vi "SigMath Class - Set FP Window Title.vi"(5 "error in (no error)":errorcluster, 7 "Application Name":string="Unknown") -> (19 "error out":errorcluster)   [LabVIEW 2020, in "SigMath.lvclass"]
uses:
  SigMath.lvclass
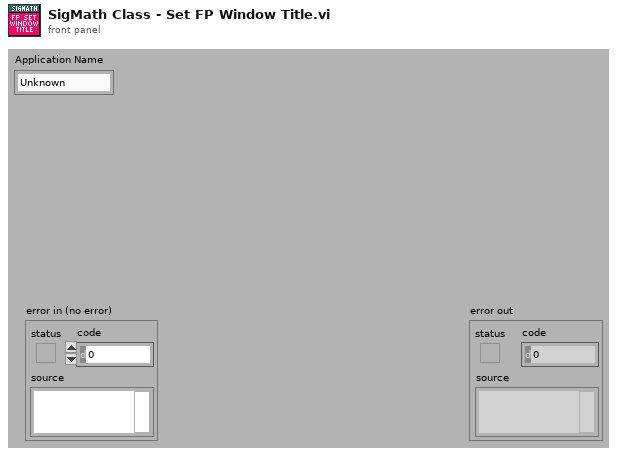
[diagram p1: front panel]
types:
  T1 = typedef "SigMath.lvclass/ClassAttributes.ctl" = cluster{"Window List":refnum<vi>[]}
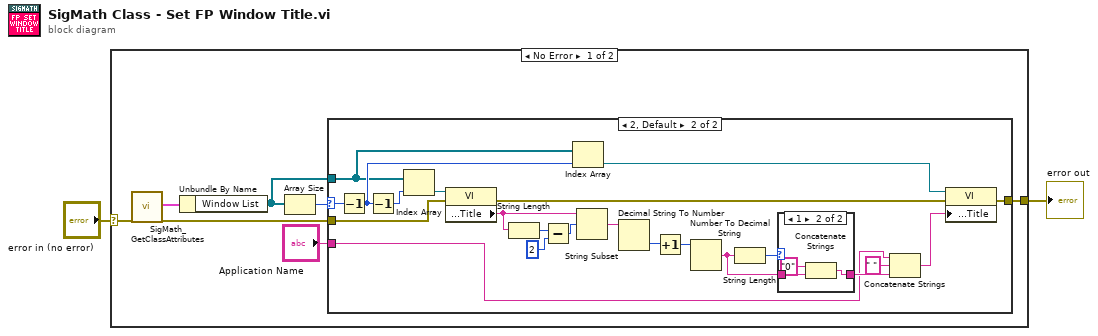
[diagram p0: block diagram]
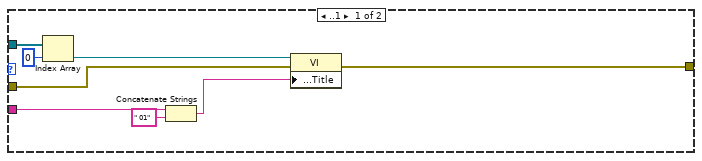
[diagram p2: hidden frame]
diagram:
  n1 = case shown="No Error" "error in (no error)" {
    selector: "error in (no error)" -> [w9 w44]
    tunnel: [w4 w44] -> w1
    frame No Error {
      n2 = call "SigMath_GetClassAttributes.vi"("error in (no error)"=w9) -> ("class attributes"=w8:T1, "error out"=w5:errorcluster)  [unwired: 15 in, 2 out]
      n3 = Unbundle By Name(w8) -> ("Window List"=w6:refnum<vi>[])
      n4 = Array Size(array=w6) -> (size(s)=w7:i32)
      n5 = case shown="2, Default" w7 {
        selector: w7 -> [_ w39]
        tunnel: w6 -> [w17 w34]
        tunnel: w5 -> [w13 w36]
        tunnel: [w14 w31] -> w4
        tunnel: "Application Name" -> [w12 w19]
        frame ..1 {
          n6 = Index Array(array=w17, index=0) -> (element=w15:refnum<vi>)
          n7 = Concatenate Strings(w12, " 01" ("string")) -> (w10:string)
          n8 = property class="VI"(reference=w15, error in=w13, "Front Panel.Title"=w10) -> (error out=w14:errorcluster)  [unwired: 1 out]
        }
        frame 2, Default {
          n9 = Decrement(x=w39) -> (x-1=w35:i32)
          n10 = Decrement(x=w35) -> (x-1=w38:i32)
          n11 = Index Array(array=w34, index=w38) -> (element=w37:refnum<vi>)
          n12 = property class="VI"(reference=w37, error in=w36) -> (error out=w33:errorcluster, "Front Panel.Title"=w30:string)  [unwired: 1 out]
          n13 = String Length(string=w30) -> (length=w29:i32)
          n14 = Subtract(x=w29, y=2) -> (x-y=w27:i32)
          n15 = Index Array(array=w34, index=w35) -> (element=w32:refnum<vi>)
          n16 = String Subset(string=w30, offset (0)=w27) -> (substring=w26:string)  [unwired: 1 in]
          n17 = Decimal String To Number(string=w26) -> (number=w25:i32)  [unwired: 2 in, 1 out]
          n18 = Increment(x=w25) -> (x+1=w24:i32)
          n19 = Number To Decimal String(number=w24) -> (decimal integer string=w22:string)  [unwired: 1 in]
          n20 = String Length(string=w22) -> (length=w23:i32)
          n21 = case shown="1" w23 {
            tunnel: [w40 w43] -> w21
            tunnel: w22 -> [w40 w42]
            frame 2, Default {
            }
            frame 1 {
              n22 = Concatenate Strings("0" ("string"), w42) -> (w43:string)
            }
          }
          n23 = Concatenate Strings(w19, " " ("string"), w21) -> (w18:string)
          n24 = property class="VI"(reference=w32, error in=w33, "Front Panel.Title"=w18) -> (error out=w31:errorcluster)  [unwired: 1 out]
        }
      }
    }
    frame Error {
    }
  }
  "error out" <- w1
